vi "Camera Setting.vi"() -> ()   [LabVIEW 2020, in "Setting Lib.lvlib"]
uses:
  Setting Lib.lvlib
  Database Lib.lvlib
panel:
  out "Last Error":string[](array[string])
  out "Over Temperature":bool
  out "Critical Temperature":bool
  out "Temperature":dbl format="%.2f"
  out "Frame Rate":dbl format="%.2f"
  out "Height":i64
  out "Width":i64
  in  "Clear Last Error":bool
  in  "Exposure Time":dbl
  in  "Offset Y":i64
  in  "Offset X":i64
  in  "Gain":i64
  in  "Close":bool
  # "Camera Settings"
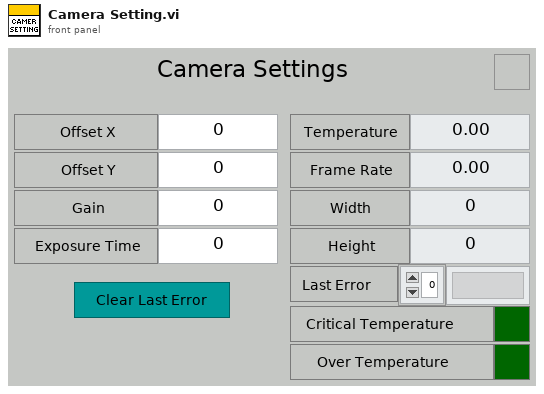
[diagram p1: front panel]
types:
  T1 = cluster{"Offset X":i64, "Offset Y":i64, "Gain":i64, "Exposure Time":dbl}
  T2 = cluster{"Offset X":i64, "Offset Y":i64, "Gain":i64, "Exposure Time":dbl}[]
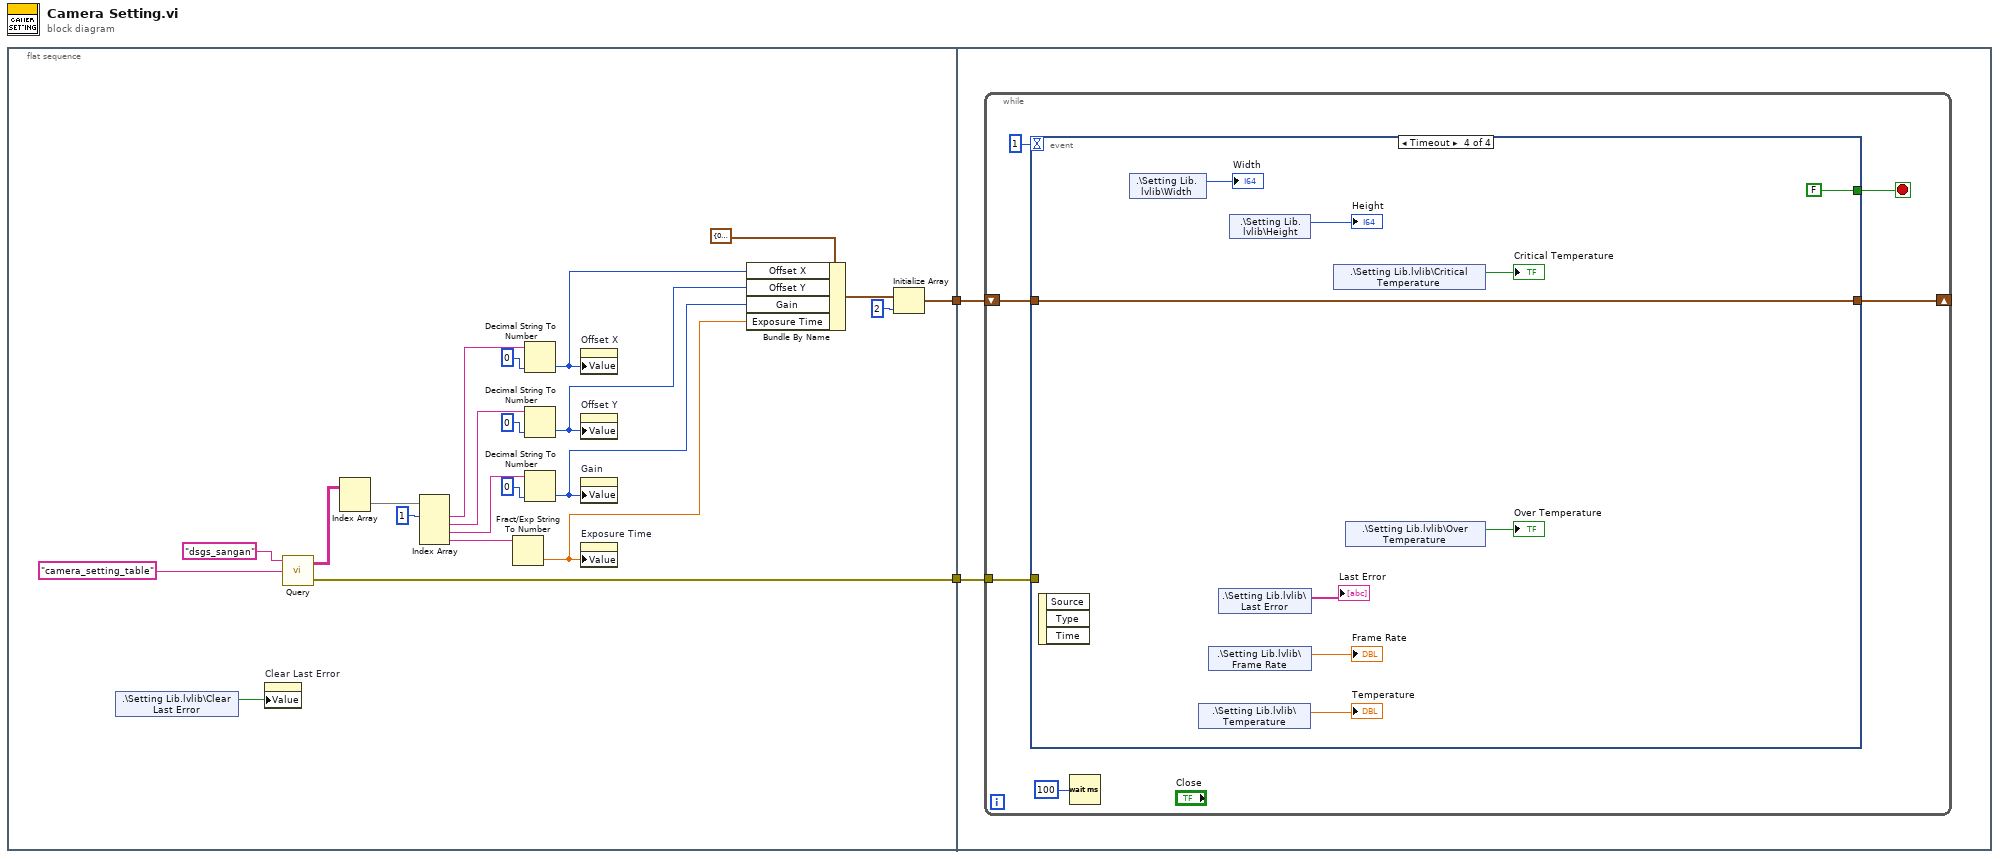
[diagram p0: block diagram]
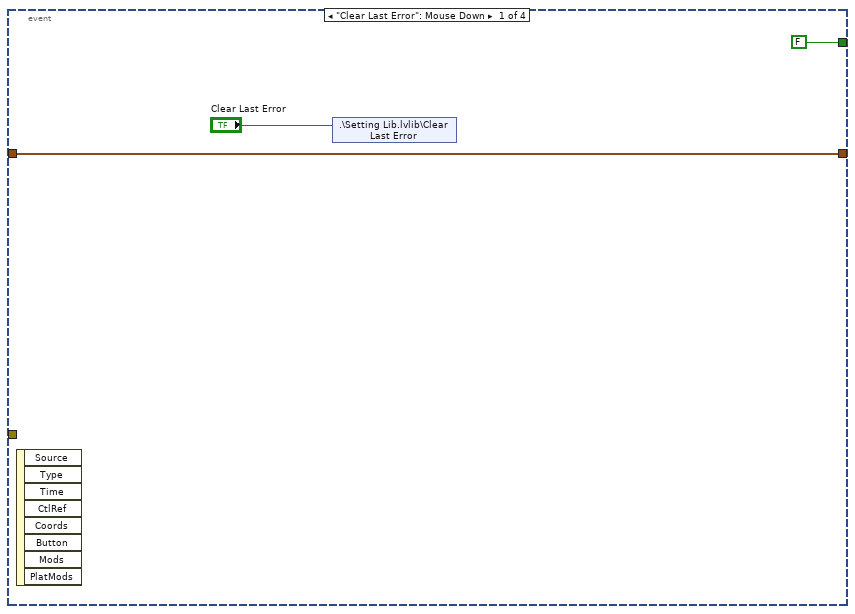
[diagram p2: hidden frame]
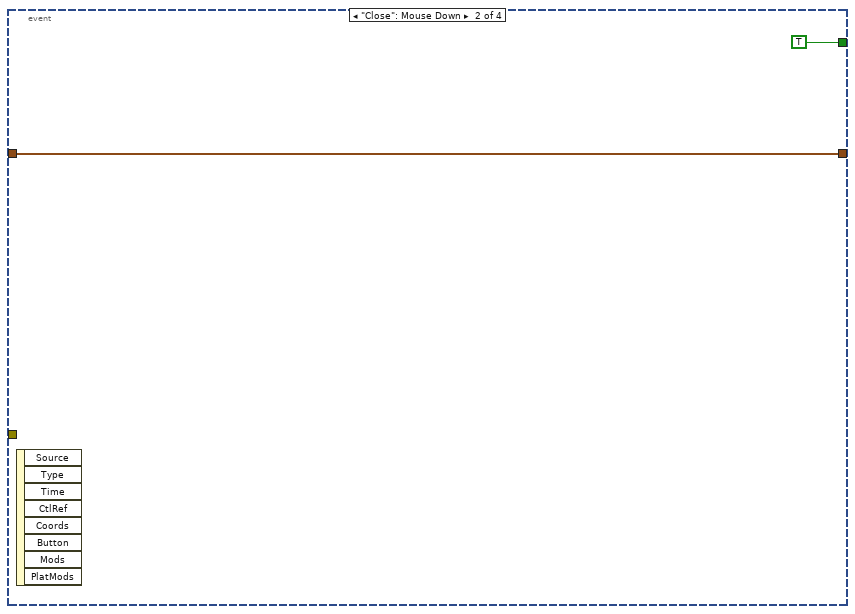
[diagram p3: hidden frame]
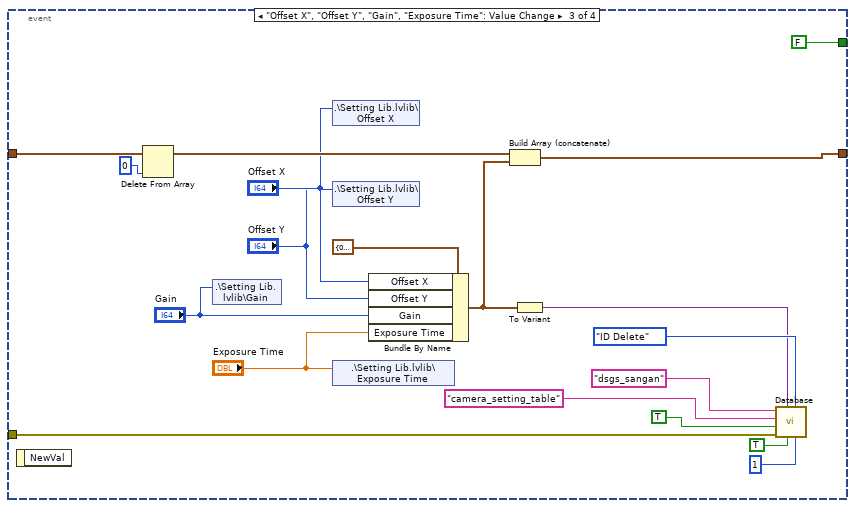
[diagram p4: hidden frame]
diagram:
  n1 = flat-sequence {
    tunnel: [w5] -> w2
    tunnel: [w4] -> w1
    tunnel: w2 -> [w26]
    tunnel: w1 -> [w25]
    frame #0 {
      n2 = shared-variable ".\\Setting Lib.lvlib\\Clear Last Error"() -> (w3:bool)  [unwired: 1 in, 1 out]
      n3 = property on="Clear Last Error" class="Bool (strict)"("Value"=w3) -> ()  [unwired: 2 in, 2 out]
      n4 = call "Query.vi"("Table Name"="camera_setting_table", "Connection Name"="dsgs_sangan") -> ("Error out"=w4:errorcluster, "data"=w14:string[][])  [unwired: 2 in]
      n5 = Index Array(array=w14) -> (element=w15:string[])  [unwired: 2 in]
      n6 = Index Array(array=w15, index #1=1 ("index")) -> (element #1=w16:string, element #2=w17:string, element #3=w18:string, element #4=w19:string)  [unwired: 3 in]
      n7 = Fract/Exp String To Number(string=w19) -> (number=w24:dbl)  [unwired: 3 in, 1 out]
      n8 = Decimal String To Number(string=w16, default (0L)=i64 0 ("default (0 I32)")) -> (number=w21:i64)  [unwired: 1 in, 1 out]
      n9 = Decimal String To Number(string=w17, default (0L)=i64 0 ("default (0 I32)")) -> (number=w22:i64)  [unwired: 1 in, 1 out]
      n10 = Decimal String To Number(string=w18, default (0L)=i64 0 ("default (0 I32)")) -> (number=w23:i64)  [unwired: 1 in, 1 out]
      n11 = property on="Offset X" class="DigNum (strict)"("Value"=w21) -> ()  [unwired: 2 in, 2 out]
      n12 = property on="Offset Y" class="DigNum (strict)"("Value"=w22) -> ()  [unwired: 2 in, 2 out]
      n13 = property on="Gain" class="DigNum (strict)"("Value"=w23) -> ()  [unwired: 2 in, 2 out]
      n14 = property on="Exposure Time" class="DigNum (strict)"("Value"=w24) -> ()  [unwired: 2 in, 2 out]
      n15 = Bundle By Name(cluster=T1 {"Offset X"=0, "Offset Y"=0, "Gain"=0, "Exposure Time"=0.0}, "Offset X"=w21, "Offset Y"=w22, "Gain"=w23, "Exposure Time"=w24) -> (w20:T1)
      n16 = Initialize Array(w20, 2 ("dimension size")) -> (w5:T2)
    }
    frame #1 {
      n17 = while {
        shift-right: [w29] -> _
        shift-left: w26 -> [w30]
        tunnel: w25 -> [w28]
        stop <- w32 stop-if-true
        n18 = event shown="[3] Timeout" {
          selector: _ -> [_ _ _ _]
          dyn-events: _ -> [_ _ _ _]
          timeout: 1 -> [_ _ _ _]
          tunnel: [FALSE TRUE FALSE FALSE] -> w32
          tunnel: w30 -> [w33 w36 w55 w58]
          tunnel: [w33 w36 w47 w58] -> w29
          tunnel: w28 -> [_ _ w43 _]
          event "Clear Last Error": Mouse Down {
            n19 = event-data() -> ()  [unwired: 1 in, 8 out]
            n20 = shared-variable ".\\Setting Lib.lvlib\\Clear Last Error"("Clear Last Error") -> ()  [unwired: 1 in, 1 out]
          }
          event "Close": Mouse Down {
            n21 = event-data() -> ()  [unwired: 1 in, 8 out]
          }
          event "Offset X", "Offset Y", "Gain", "Exposure Time": Value Change {
            n22 = event-data() -> ()  [unwired: 1 in, 1 out]
            n23 = Delete From Array(array=w55, index=0) -> (array with subset deleted=w54:T2)  [unwired: 1 in, 1 out]
            n24 = shared-variable ".\\Setting Lib.lvlib\\Gain"("Gain") -> ()  [unwired: 1 in, 1 out]
            n25 = shared-variable ".\\Setting Lib.lvlib\\Offset X"("Offset X") -> ()  [unwired: 1 in, 1 out]
            n26 = shared-variable ".\\Setting Lib.lvlib\\Offset Y"("Offset Y") -> ()  [unwired: 1 in, 1 out]
            n27 = shared-variable ".\\Setting Lib.lvlib\\Exposure Time"("Exposure Time") -> ()  [unwired: 1 in, 1 out]
            n28 = Bundle By Name(cluster=T1 {"Offset X"=0, "Offset Y"=0, "Gain"=0, "Exposure Time"=0.0}, "Offset X"="Offset X", "Offset Y"="Offset Y", "Gain"="Gain", "Exposure Time"="Exposure Time") -> (w39:T1)
            n29 = Build Array (concatenate)(w54, w39) -> (w47:T2)
            n30 = To Variant(anything=w39) -> (Variant=w38:variant)
            n31 = call "Database.vi"("Maximum Row"=1, "Enum"=enum16{"ID Delete", "Time Delete"}."ID Delete", "Delete row?"=TRUE, "Data"=w38, "Error in"=w43, "Auto Increment ID?"=TRUE, "Table"="camera_setting_table", "Connection"="dsgs_sangan") -> ()  [unwired: 3 in, 1 out]
          }
          event Timeout {
            n32 = event-data() -> ()  [unwired: 1 in, 3 out]
            n33 = shared-variable ".\\Setting Lib.lvlib\\Width"() -> (→"Width":i64)  [unwired: 1 in, 1 out]
            n34 = shared-variable ".\\Setting Lib.lvlib\\Temperature"() -> (→"Temperature":dbl)  [unwired: 1 in, 1 out]
            n35 = shared-variable ".\\Setting Lib.lvlib\\Frame Rate"() -> (→"Frame Rate":dbl)  [unwired: 1 in, 1 out]
            n36 = shared-variable ".\\Setting Lib.lvlib\\Last Error"() -> (→"Last Error":string[])  [unwired: 1 in, 1 out]
            n37 = shared-variable ".\\Setting Lib.lvlib\\Height"() -> (→"Height":i64)  [unwired: 1 in, 1 out]
            n38 = shared-variable ".\\Setting Lib.lvlib\\Critical Temperature"() -> (→"Critical Temperature":bool)  [unwired: 1 in, 1 out]
            n39 = shared-variable ".\\Setting Lib.lvlib\\Over Temperature"() -> (→"Over Temperature":bool)  [unwired: 1 in, 1 out]
          }
        }
        n40 = Wait (ms)(milliseconds to wait=u32 100) -> ()  [unwired: 1 out]
      }
    }
  }
